vi "TEST_SendSTR2Var_TEST.vi"() -> ()   [LabVIEW 2009, in "MoAgSy_TEST.lvlib"]
uses:
  MoAgSy_TEST/MoAgSy_TEST.lvlib
  MoAgSy_Message/MoAgSy_Message.lvclass
  MoAgSy_Factory/MoAgSy_Factory.lvclass
  MoAgSy_TEST/AgentChildTest/AgentChildTest.lvclass
  MoAgSy_AgentBase/MoAgSy_AgentBase.lvclass
  HGF_BaseClasses/HGF_Factory/HGF_Factory.lvclass
  <vilib>/lvdsc/NI_DSC.lvlib
panel:
  in  "Shared Variable Control":refnum<k21>="\\\\localhost\\HGFObj_2009-12-15_12:29:45,794\\TestHost"
  out "Host var String":string
  out "time diff":dbl
  in  "Agent/\nAgentChildTest":bool=TRUE
  out "objectName":string
  out "reply addressee":string
  out "Message":string
  in  "message type":enum16{"travel request", "false"}(ring)
  in  "message":string
  out "reply value\n change":bool
  in  "request reply":bool=TRUE
  in  "send continous":bool
  in  "send one":bool
  in  "milliseconds to wait":u32
  in  "randomized?":bool
  in  "stop":bool
  in  "type":enum16{"mobile Agent", "Visitor", "Message"}(ring)
  in  "addressee":string="TestHost"
  out "Submitted Object":string
  # "Select shared Variable \nbefore you start the Test"
  # "Reply"
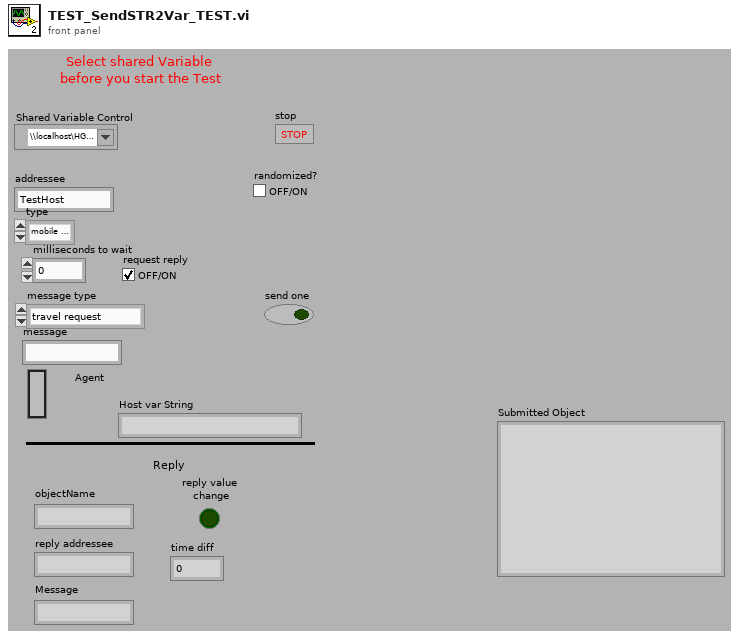
[diagram p1: front panel]
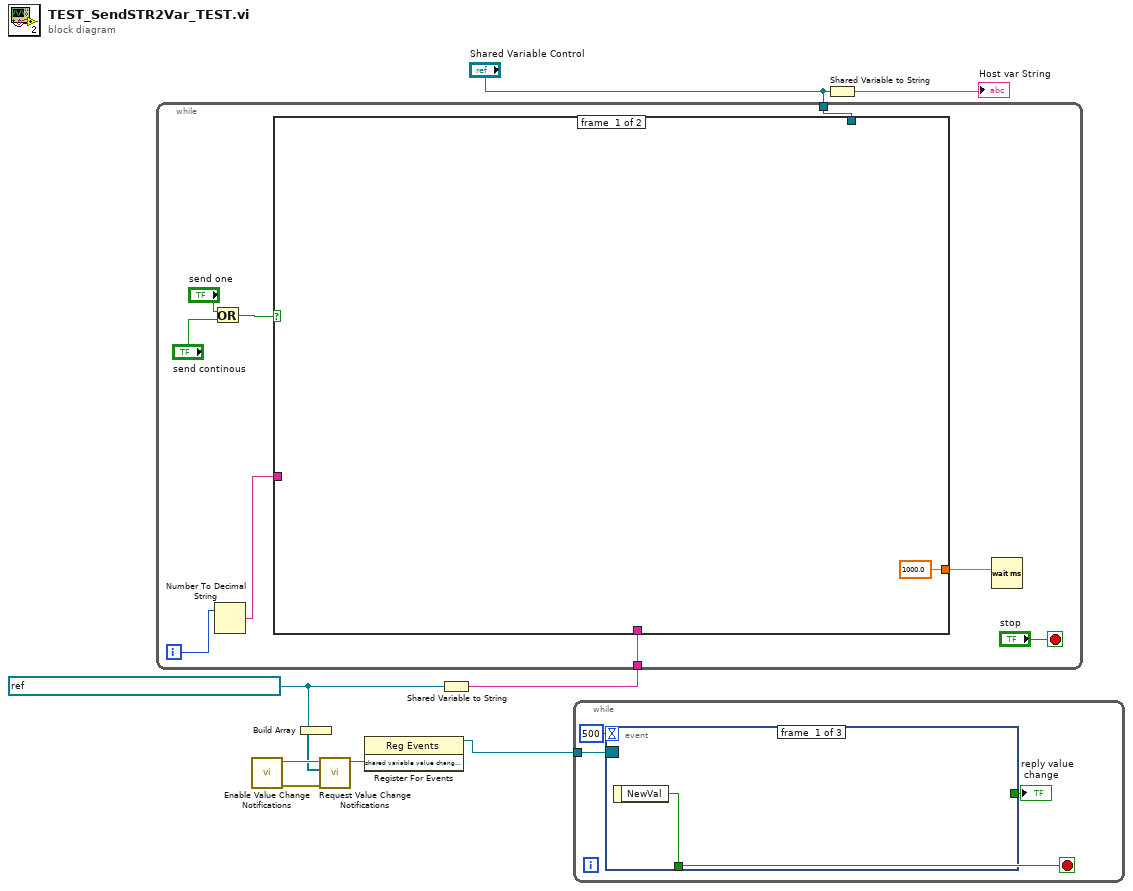
[diagram p0: block diagram]
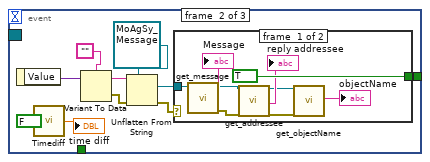
[diagram p2: hidden frame]
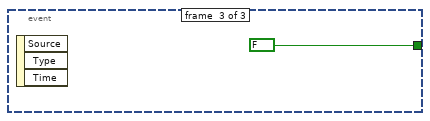
[diagram p4: hidden frame]
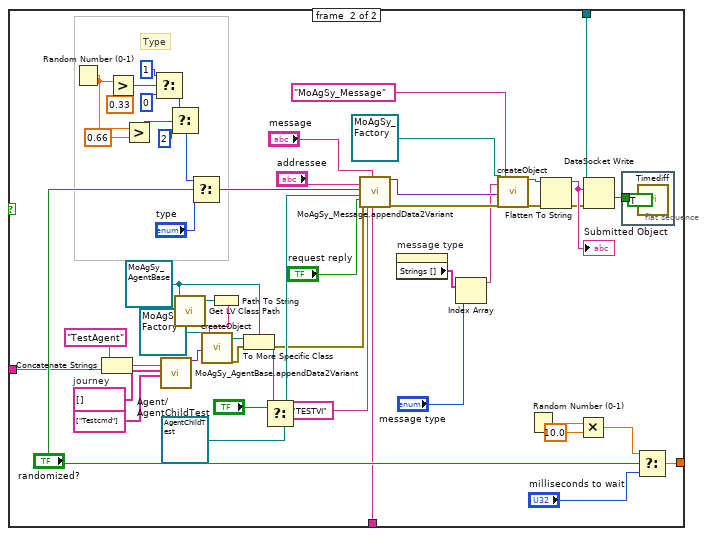
[diagram p5: hidden frame]
diagram:
  w6 = refnum<k21> "\\\\My Computer\\MoAgSy_TEST\\Reply Variable"
  n1 = call <vilib>:"Enable Value Change Notifications.vi"() -> ("error out"=w7:errorcluster, "shared variable value change notification"=w8:refnum<user-event>)  [unwired: 1 in, 9 out]
  n2 = Build Array(w6) -> (w5:refnum<k21>[])
  n3 = call <vilib>:"Request Value Change Notifications.vi"("error in (no error)"=w7, "shared variables"=w5, "notification refnum"=w8) -> ("shared variable value change notification"=w4:refnum<user-event>)  [unwired: 1 in, 7 out]
  n4 = register-events(w4) -> (reference out=w3:refnum<event-registration>)  [unwired: 2 in, 1 out]
  n5 = Shared Variable to String(1:w6) -> (0:w9:string)
  n6 = while {
    tunnel: "Shared Variable Control" -> [w16]
    tunnel: w9 -> [w12]
    i -> [w11]
    stop <- "stop" stop-if-true
    n7 = Or(x="send one", y="send continous") -> (x .or. y?=w15:bool)
    n8 = Number To Decimal String(number=w11) -> (decimal integer string=w10:string)  [unwired: 1 out]
    n9 = case shown="True" w15 {
      tunnel: [1000.0 ("milliseconds to wait") w46] -> w17
      tunnel: w16 -> [_ w44]
      tunnel: w12 -> [_ w42]
      tunnel: w10 -> [_ w20]
      frame #0 {
      }
      frame #1 {
        w25 = string[] []  # journey
        w29 = refnum<class "MoAgSy_AgentBase.lvclass"> refnum ("MoAgSy.lvlib:MoAgSy_Base.lvlib:MoAgSy_AgentBase.lvclass")
        # "Type"
        n10 = Random Number (0-1)() -> (number: 0 to 1=w57:dbl)
        n11 = Concatenate Strings("TestAgent" ("Agent name"), w20) -> (w21:string)
        n12 = Greater?(x=w57, y=0.33) -> (0:w55:bool)
        n13 = Greater?(x=w57, y=0.66) -> (0:w51:bool)
        n14 = Select(t=u16 1, s=w55, f=u16 0) -> (s? t:f=w52:u16)
        n15 = call "MoAgSy_AgentBase.appendData2Variant.vi"("Agent name"=w21, "journey"=w25, "Command names"=string[] ["Testcmd"]) -> ("dup init"=w27:variant)  [unwired: 4 in, 12 out]
        n16 = Select(t=w52, s=w51, f=u16 2) -> (s? t:f=w49:u16)
        n17 = call <vilib>:"Get LV Class Path.vi"("object"=w29) -> ("class path"=w32:path)  [unwired: 1 in, 9 out]
        n18 = Select(t=w49, s="randomized?", f="type") -> (s? t:f=w61:u16)
        n19 = Path To String(path=w32) -> (string=w31:string)
        n20 = call "createObject.vi"("HGF_Factory"=refnum<class "MoAgSy_Factory.lvclass"> refnum ("MoAgSy.lvlib:MoAgSy_Factory.lvclass"), "initializationData"=w27, "className"=w31) -> ("HGF_Object"=w30:refnum<class "HGF_Factory.lvclass">, "error out"=w23:errorcluster)  [unwired: 2 in, 13 out]
        n21 = To More Specific Class(target class=w29, reference=w30, error in=w23) -> (specific class reference=w28:refnum<class "MoAgSy_AgentBase.lvclass">, error out=w22:errorcluster)
        n22 = Select(t=w28, s="Agent/\nAgentChildTest", f=refnum<class "AgentChildTest.lvclass"> refnum ("MoAgSy_TEST.lvlib:AgentChildTest.lvclass")) -> (s? t:f=w36:refnum<class "MoAgSy_AgentBase.lvclass">)
        n23 = call "MoAgSy_Message.appendData2Variant.vi"("addressee"="addressee", "type"=w61, "Object"=w36, "request reply"="request reply", "error in"=w22, "sender"="TESTVI", "message"="message", "reply to"=w42) -> ("dup_initData"=w70:variant, "error out"=w69:errorcluster)  [unwired: 3 in, 7 out]
        n24 = property on="message type" class="Enum (strict)"() -> ("Strings []"=w41:string[])  [unwired: 2 in, 2 out]
        n25 = Index Array(array=w41, index="message type") -> (element=w39:string)
        n26 = call "createObject.vi"("HGF_Factory"=refnum<class "MoAgSy_Factory.lvclass"> refnum ("MoAgSy.lvlib:MoAgSy_Factory.lvclass"), "objectName"=w39, "initializationData"=w70, "error in (no error)"=w69, "className"="MoAgSy_Message") -> ("HGF_Object"=w68:refnum<class "HGF_Factory.lvclass">, "error out"=w66:errorcluster)  [unwired: 13 out]
        n27 = Random Number (0-1)() -> (number: 0 to 1=w63:dbl)
        n28 = Flatten To String(anything=w68, error in (no error)=w66) -> (data string=w67:string, error out=w65:errorcluster)  [unwired: 3 out]
        "Submitted Object" <- w67
        n29 = Multiply(x=w63, y=10.0) -> (x*y=w48:dbl)
        n30 = DataSocket Write(8:w65, 10:w67, 11:w44) -> (1:w34:bool)  [unwired: 3 out]
        n31 = flat-sequence {
          tunnel: w34 -> [_]
          frame #0 {
            n32 = call "Timediff.vi"("Start/Stop"=TRUE) -> ()  [unwired: 1 out]
          }
        }
        n33 = Select(t=w48, s="randomized?", f="milliseconds to wait") -> (s? t:f=w46:dbl)
      }
    }
    n34 = Wait (ms)(milliseconds to wait=w17) -> ()  [unwired: 1 out]
  }
  n35 = while {
    tunnel: w3 -> [w77]
    stop <- w76 stop-if-true
    n36 = event shown="[1] <shared variable value change notification>: User Event" {
      selector: w77 -> [_ _ _]
      dyn-events: _ -> [_ _ _]
      timeout: 500 -> [_ _ _]
      tunnel: [w78 _ _] -> w76
      tunnel: [_ w88 FALSE] -> w74
      event #0 {
        n37 = event-data() -> ("NewVal"=w78:bool)  [unwired: 1 out]
      }
      event #1 {
        n38 = event-data() -> ("Value"=w87:variant)  [unwired: 1 out]
        n39 = call "Timediff.vi"("Start/Stop"=FALSE) -> ("x-y"=→"time diff":dbl)
        n40 = Variant To Data(Variant=w87, type="") -> (error out=w82:errorcluster, data=w85:string)  [unwired: 1 in]
        n41 = Unflatten From String(type=refnum<class "MoAgSy_Message.lvclass"> refnum ("MoAgSy.lvlib:MoAgSy_Message.lvclass"), binary string=w85, error in (no error)=w82) -> (value=w83:refnum<class "MoAgSy_Message.lvclass">, error out=w81:errorcluster)  [unwired: 3 out]
        n42 = case shown="No Error" w81 {
          tunnel: [TRUE _] -> w88
          tunnel: w83 -> [w96 _]
          frame #0 {
            n43 = call "get_message.vi"("MoAgSy_Message.lvclass in"=w96) -> ("error out"=w90:errorcluster, "Message"=→"Message":string, "MoAgSy_Message.lvclass out"=w94:refnum<class "MoAgSy_Message.lvclass">)  [unwired: 1 in, 7 out]
            n44 = call "get_addressee.vi"("MoAgSy_Message in"=w94, "error in (no error)"=w90) -> ("MoAgSy_Message out"=w92:refnum<class "MoAgSy_Message.lvclass">, "addressee"=→"reply addressee":string, "error out"=w89:errorcluster)  [unwired: 15 out]
            n45 = call "get_objectName.vi"("HGF_Factory"=w92, "error in (no error)"=w89) -> ("objectName"=→"objectName":string)  [unwired: 17 out]
          }
          frame #1 {
          }
        }
      }
      event #2 {
        n46 = event-data() -> ()  [unwired: 4 out]
      }
    }
    "reply value\n change" <- w74
  }
  n47 = Shared Variable to String(1:"Shared Variable Control") -> (0:→"Host var String":string)
